vi "扫描.vi"   [LabVIEW 2019]
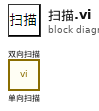
[diagram p0: block diagram]
diagram:
  n1 = call "单向扫描.vi"() -> ()  [unwired: 9 in, 3 out]
  n2 = call "双向扫描.vi"() -> ()  [unwired: 8 in, 4 out]
